vi "TestReport_resizeImages.vi"(8 "error in (no error)":errorcluster, 11 "TestReport_data in":T1) -> (0 "error out":errorcluster, 3 "TestReport_data out":T1)   [LabVIEW 2016]
uses:
  TestReport_data.ctl
  <vilib>/Utility/NIReport.llb/NI_report.lvclass
  WorReport_imageData.ctl
  WorReport_tableData.ctl
  <vilib>/Utility/miscctls.llb/LVBoundsTypeDef.ctl
panel:
  in  "Altura":sgl=372.0
  out "Image":picture
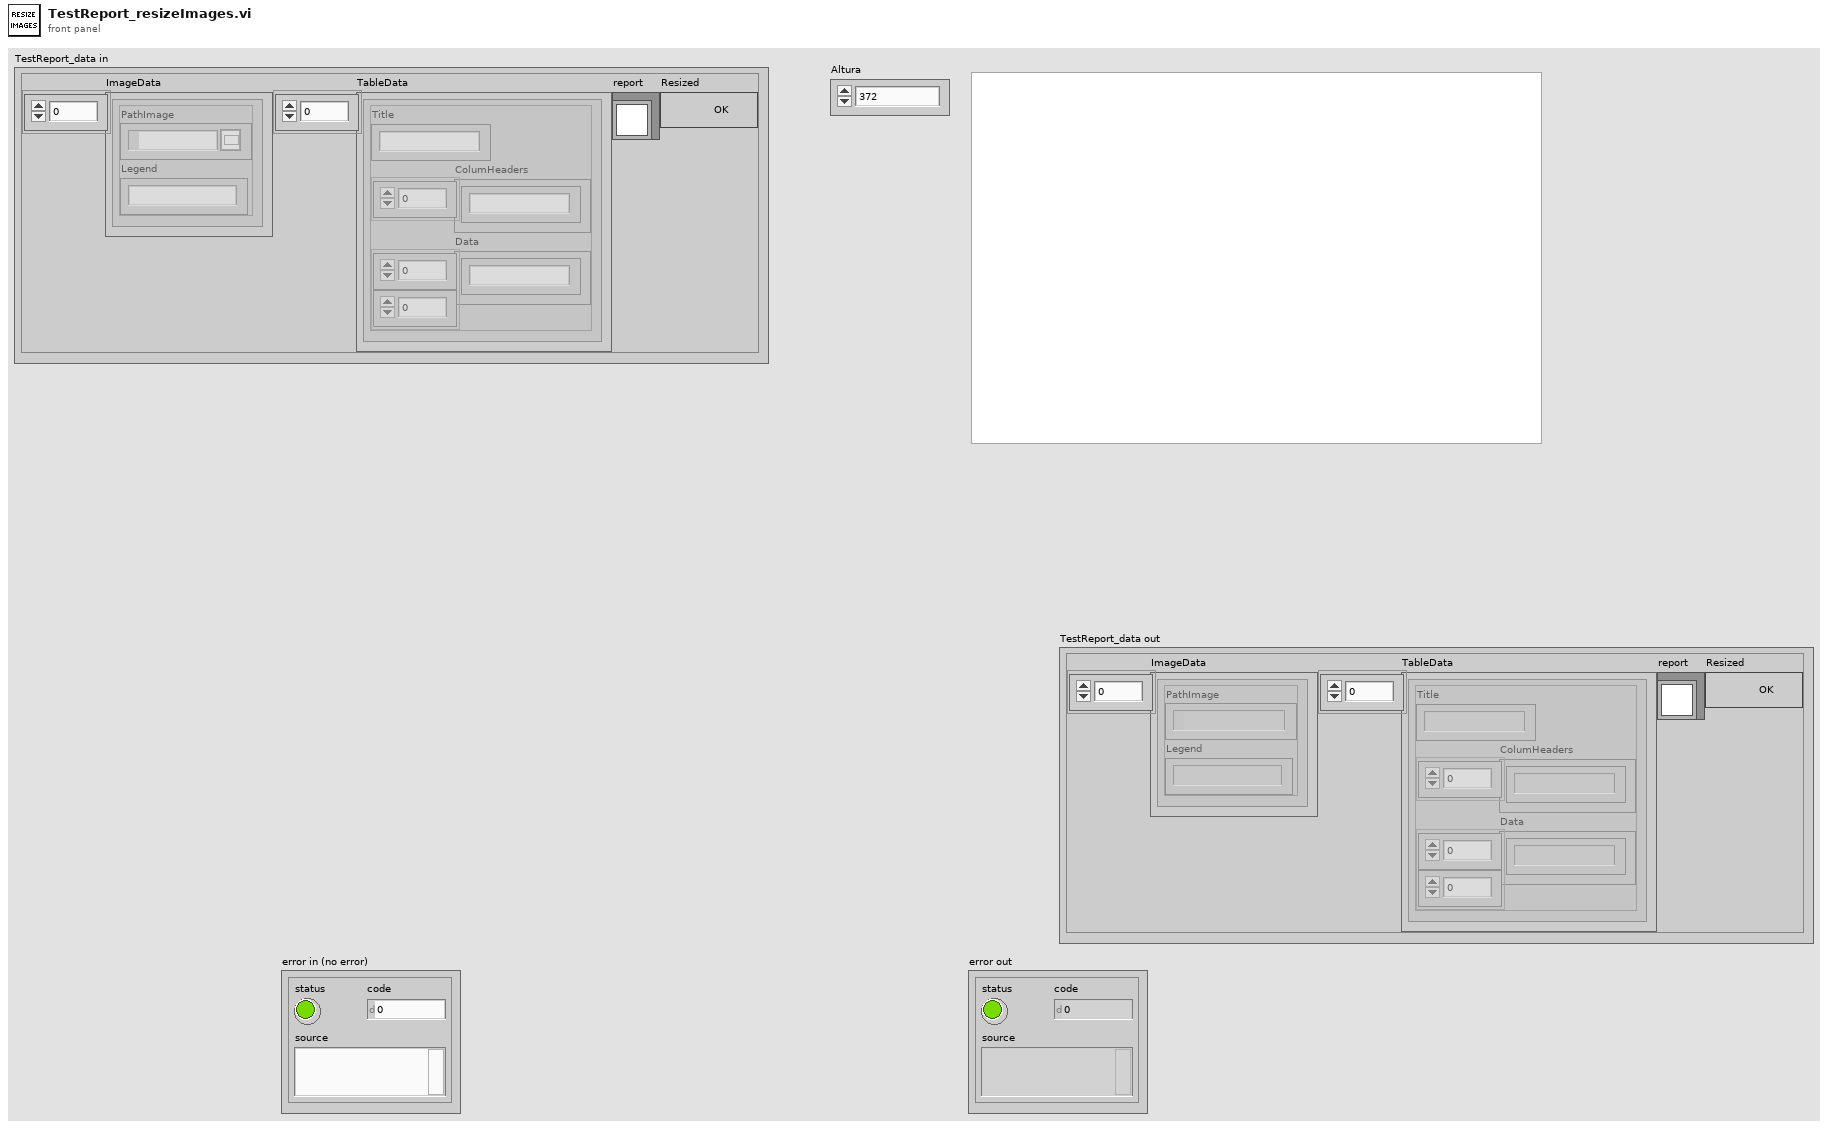
[diagram p1: front panel]
types:
  T1 = typedef "TestReport_data.ctl" = cluster{"ImageData":T2[], "TableData":T3[], "report":refnum<class "NI_report.lvclass">, "Resized":bool}
  T2 = typedef "WorReport_imageData.ctl" = cluster{"PathImage":path, "Legend":string}
  T3 = typedef "WorReport_tableData.ctl" = cluster{"Title":string, "ColumHeaders":string[], "Data":string[][]}
  T4 = typedef "LVBoundsTypeDef.ctl" = cluster{"Width":u32, "Height":u32}
  T5 = typedef "imagedata.ctl" = cluster{"image type":i32, "image depth":i32, "image":u8[], "mask":u8[], "colors":u32[], "Rectangle":cluster{"left":i16, "top":i16, "right":i16, "bottom":i16}}
  T6 = cluster{"left":i16, "top":i16, "right":i16, "bottom":i16}
  T7 = cluster{"left":sgl, "top":sgl, "right":sgl, "bottom":sgl}
  T8 = cluster{"left":u32, "top":u32, "right":u32, "bottom":u32}
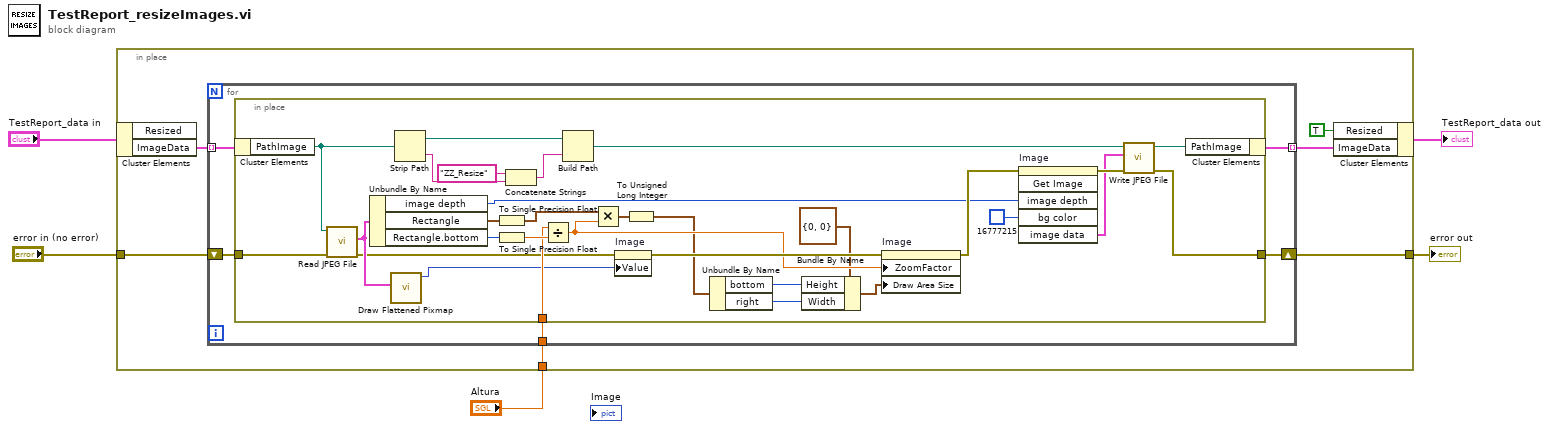
[diagram p0: block diagram]
diagram:
  n1 = in-place {
    in-place-border: "error in (no error)" -> [w10]
    in-place-border: [w9] -> w4
    in-place-border: "Altura" -> [w7]
    n2 = in-place-cluster #1("TestReport_data in") -> ("ImageData"=w11:T2[])  [unwired: 1 out]
    n3 = for {
      tunnel: w11 -> [w16] mode=indexing
      tunnel: [w13] -> w8 mode=indexing
      shift-right: [w14] -> w9
      shift-left: w10 -> [w15]
      tunnel: w7 -> [w12]
      n4 = in-place {
        in-place-border: w15 -> [w46]
        in-place-border: [w29] -> w14
        in-place-border: w12 -> [w42]
        n5 = in-place-cluster #2(w16) -> ("PathImage"=w37:path)
        n6 = call <vilib>:"Read JPEG File.vi"("error in (no error)"=w46, "path to JPEG file"=w37) -> ("error out"=w40:errorcluster, "image data"=w45:T5)  [unwired: 7 in, 1 out]
        n7 = Unbundle By Name(w45) -> ("image depth"=w27:i32, "Rectangle"=w18:T6, "Rectangle.bottom"=w44:i16)
        n8 = call <vilib>:"Draw Flattened Pixmap.vi"("image data"=w45) -> ("new picture"=w41:picture)  [unwired: 8 in]
        n9 = Strip Path(path=w37) -> (stripped path=w34:path, name=w36:string)
        n10 = To Single Precision Float(number=w18) -> (single precision float=w17:T7)
        n11 = To Single Precision Float(number=w44) -> (single precision float=w43:sgl)
        n12 = Concatenate Strings("ZZ_Resize" ("string"), w36) -> (w33:string)
        n13 = Divide(x=w42, y=w43) -> (x/y=w38:sgl)
        n14 = Build Path(base path=w34, name or relative path=w33) -> (appended path=w32:path)
        n15 = Multiply(x=w17, y=w38) -> (x*y=w30:T7)
        n16 = property on="Image" class="Pict"(error in=w40, "Value"=w41) -> (error out=w39:errorcluster)  [unwired: 1 in, 1 out]
        n17 = To Unsigned Long Integer(number=w30) -> (unsigned 32bit integer=w23:T8)
        n18 = Unbundle By Name(w23) -> ("bottom"=w21:u32, "right"=w20:u32)
        n19 = Bundle By Name(cluster=T4 {"Width"=0, "Height"=0} ("Draw Area Size"), "Height"=w21, "Width"=w20) -> (w19:T4)
        n20 = property on="Image" class="Pict"(error in=w39, "ZoomFactor"=w38, "Draw Area Size"=w19) -> (error out=w28:errorcluster)  [unwired: 1 in, 1 out]
        n21 = invoke on="Image" class="Pict" method="Get Image"(error in=w28, "image depth"=w27, "bg color"=u32 16777215) -> (error out=w26:errorcluster, "image data"=w25:T5)  [unwired: 3 in, 4 out]
        n22 = call <vilib>:"Write JPEG File.vi"("error in (no error)"=w26, "image data"=w25, "path to JPEG file"=w32) -> ("error out"=w29:errorcluster, "path"=w31:path)  [unwired: 7 in]
        n23 = in-place-cluster #2("PathImage"=w31) -> (w13:T2)
      }
    }
    n24 = in-place-cluster #1("Resized"=TRUE, "ImageData"=w8) -> (→"TestReport_data out":T1)
  }
  "error out" <- w4
